vi "SPI Open Channel.vi"(8 "error in (no error)":errorcluster, 10 "handle":u32 format="%08x", 11 "index":u32) -> (0 "error out":errorcluster, 3 "handle out":u32 format="%08x")   [LabVIEW 2018, in "libMPSSE-SPI.lvlib"]
doc: "FTDI_API FT_STATUS SPI_OpenChannel(uint32 index, FT_HANDLE *handle);"
uses:
  libMPSSE-SPI.lvlib
  dll/libMPSSE.dll
panel:
  out "function return":u32
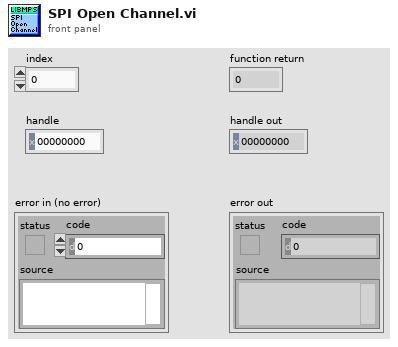
[diagram p1: front panel]
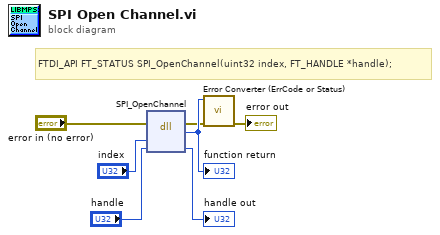
[diagram p0: block diagram]
diagram:
  # "FTDI_API FT_STATUS SPI_OpenChannel(uint32 index, FT_HANDLE *handle);"
  n1 = dll-call lib="D:/LABVIEW/Examples - 32bit/FTDI/libMPSSE-SPI-LabVIEW-master/dll/libMPSSE.*" fn="SPI_OpenChannel"(error in="error in (no error)", "index"="index", "handle"="handle") -> (error out=w2:errorcluster, "return type"=w7:u32, "handle"=→"handle out":u32)  [unwired: 3 in, 1 out]
  "function return" <- w7
  n2 = call "Error Converter (ErrCode or Status).vi"("error in (no error)"=w2, "error code"=w7) -> ("error out"=→"error out":errorcluster)  [unwired: 9 in]
